vi "RT Data processing loop.vi"(9 "Data":T1={"Parameters"={"FPGA Ref"=refnum, "data stream"={"data writer name"="error writer", "NS write buffer size"=16, "NS Buffer length"=0}, "FIFO Depth"=0, "Channel controls"={"FIFO channel count"=0, "active indices"=[], "active channels"=0, "channelScaling"=[], "scanivalveCount"=0, "channels"=[]}, "safetyChannels"={"oilP"=0, "airP"=0, "water"=0, "channelLimits"=[]}, "speedChannel"=0, "maxSpeedLimit"=0.0, "Torque"={"fixedOffset"=0.0, "filter"=FALSE, "fallingEdge"=FALSE, "swapEncoders"=FALSE}}, "Variables"={"Intermediary buffer"=[], "buffer position"=0, "write loop counter"=0, "NS write trigger"=0, "NS Connection status"=FALSE, "waiting for NS"=FALSE, "labAmbient"={"pressure"=0.0, "temperature"=0.0}, "scanivalvePorts"=[], "scanivalvePressures"=[], "data stream"="", "activeChannelLimitIndex"=[], "runningSpeedLimit"=0.0, "speedChannelIndex"=0, "Interlocks"={"gearboxOil"=FALSE, "bearingOil"=FALSE, "gearboxAir"=FALSE}, "interlockChannels"={"gearboxOil"=0, "bearingOil"=0, "air"=0}, "limitStates"=[]}}, 11 "RT Queues":T8) -> ()   [LabVIEW 2018]
uses:
  Type Defs/Queues cluster.ctl
  ICL-LabVIEW_General/Message Scheduler/message scheduler.lvclass
  Type Defs/Data processing loop data.ctl
  Type Defs/FPGA reference.ctl
  PC/type defs/channelControl.ctl
  Type Defs/channelScalingTypes.ctl
  Type Defs/scalingMethods.ctl
  ICL-LabVIEW_General/data channels/parent class/Data Channel.lvclass
  PC/type defs/channelLimitControl.ctl
  PC/type defs/limitActions.ctl
  ICL-LabVIEW_General/data channels/parent class/Data Channel.lvclass/Data Channel.ctl
  <vilib>/dex/Flush And Wait Empty Condition.ctl
  Queue VIs/De-queue RT data element.vi
  Queue VIs/En-queue RT data element.vi
  Queue VIs/En-queue RT FIFO element.vi
  <vilib>/Utility/error.llb/Error Cluster From Error Code.vi
  <vilib>/rvi/errors/niLvFpgaAdjustHostInterfaceError.vi
  Queue VIs/Close RT data queue.vi
  <vilib>/rvi/interface/nirviReadWriteControl/nirviReadWriteControl.xnode
  FPGA Bitfiles/CompressorRigV2_CompressorFPGA_FPGAMainV3_7sPRekuravM.lvbitx
  NiFpgaLv.dll
panel:
  out "# elements in queue":i32
  out "Iteration Duration":i64[](array[numeric]) caption="Iteration Duration (max 10)"
  out "Processor resources low":bool
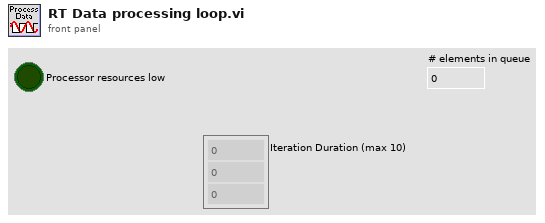
[diagram p1: front panel]
types:
  T1 = typedef "Data processing loop data.ctl" = cluster{"Parameters":cluster{"FPGA Ref":T2, "data stream":cluster{"data writer name":string, "NS write buffer size":i32, "NS Buffer length":u32}, "FIFO Depth":u32, "Channel controls":cluster{"FIFO channel count":i32, "active indices":i16[], "active channels":i32, "channelScaling":T3[], "scanivalveCount":i32, "channels":refnum<class "Data Channel.lvclass">[]}, "safetyChannels":cluster{"oilP":u16, "airP":u16, "water":u16, "channelLimits":T6[]}, "speedChannel":i32, "maxSpeedLimit":dbl, "Torque":cluster{"fixedOffset":dbl, "filter":bool, "fallingEdge":bool, "swapEncoders":bool}}, "Variables":cluster{"Intermediary buffer":dbl[][], "buffer position":u32, "write loop counter":u16, "NS write trigger":u32, "NS Connection status":bool, "waiting for NS":bool, "labAmbient":cluster{"pressure":dbl, "temperature":dbl}, "scanivalvePorts":u16[], "scanivalvePressures":dbl[], "data stream":refnum<k21>, "activeChannelLimitIndex":u16[], "runningSpeedLimit":dbl, "speedChannelIndex":i32, "Interlocks":cluster{"gearboxOil":bool, "bearingOil":bool, "gearboxAir":bool}, "interlockChannels":cluster{"gearboxOil":i32, "bearingOil":i32, "air":i32}, "limitStates":cluster{"warn":bool, "alarm":bool}[]}}
  T2 = typedef "FPGA reference.ctl" = refnum<k20>
  T3 = typedef "channelControl.ctl" = cluster{"index":u16, "active":bool, "channelType":T4, "module":u16, "terminal":u16, "channelName":string, "scalingMethod":T5, "scalingParameters":dbl[], "scaledUnits":string, "tempOffset":dbl}
  T4 = typedef "channelScalingTypes.ctl" = enum16{"calculation", "measurement", "scanivalve", "output", "digital"}
  T5 = typedef "scalingMethods.ctl" = enum16{"none", "linear", "thermocouple", "polynomial", "encoder", "RTD"}
  T6 = typedef "channelLimitControl.ctl" = cluster{"channelID":u16, "Enabled":bool, "warnValue":dbl, "limitValue":dbl, "Invert":bool, "limitAction":T7}
  T7 = typedef "limitActions.ctl" = enum16{"stop", "shutdown", "ignore"}
  T8 = typedef "Queues cluster.ctl" = cluster{"RT Message":refnum<queue>, "RT Comms":refnum<queue>, "RT Data":refnum<queue>, "RT FIFO":refnum<queue>, "message scheduler":refnum<class "message scheduler.lvclass">}
  T9 = typedef "Flush And Wait Empty Condition.ctl" = u8
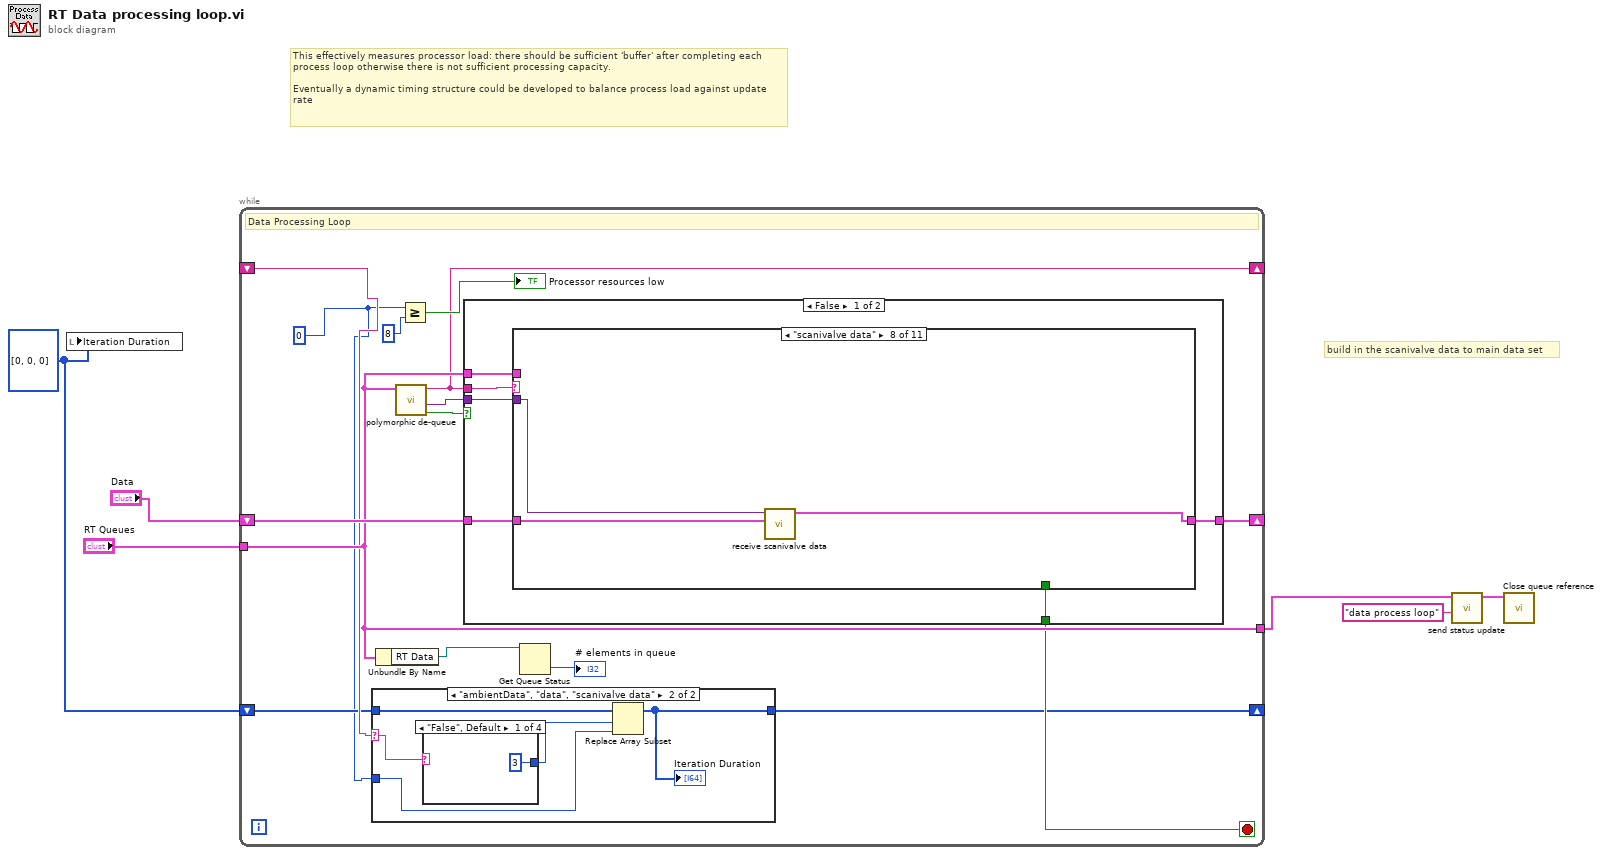
[diagram p0: block diagram]
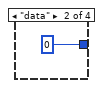
[diagram p3: hidden frame]
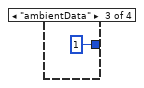
[diagram p4: hidden frame]
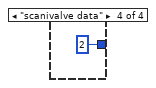
[diagram p5: hidden frame]
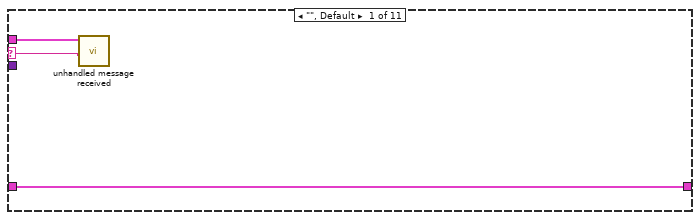
[diagram p6: hidden frame]
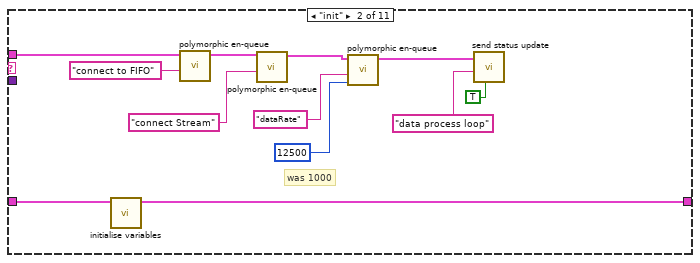
[diagram p7: hidden frame]
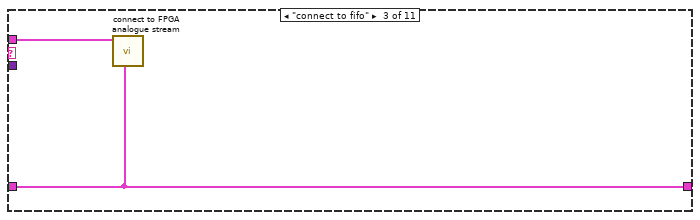
[diagram p8: hidden frame]
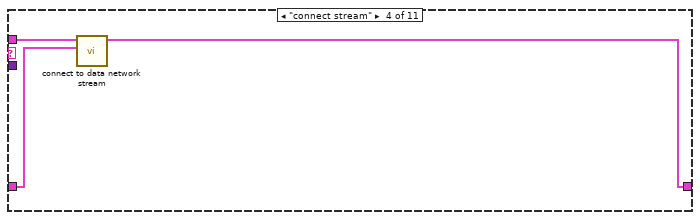
[diagram p9: hidden frame]
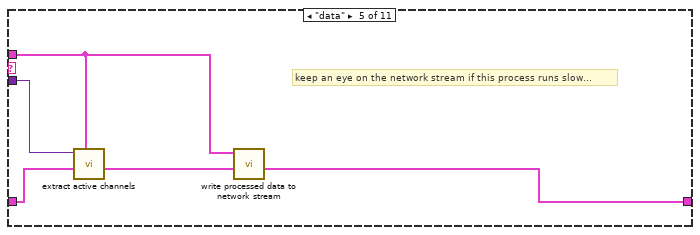
[diagram p10: hidden frame]
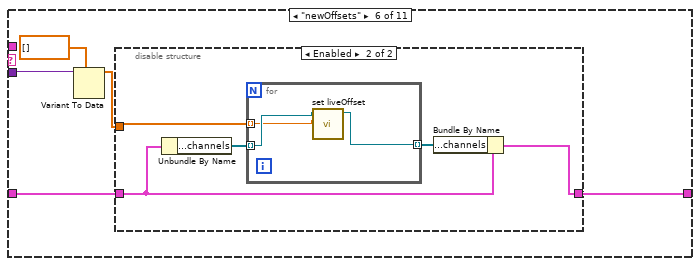
[diagram p11: hidden frame]
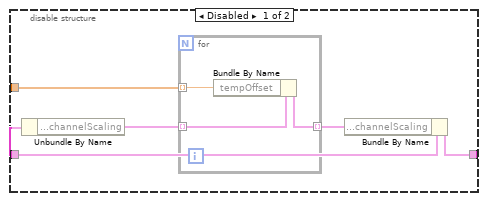
[diagram p12: hidden frame]
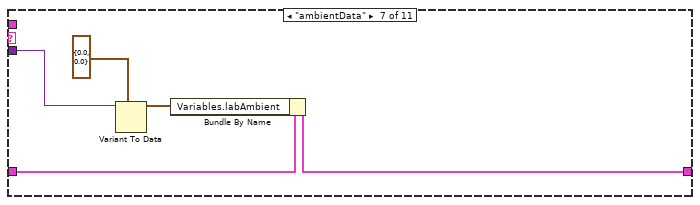
[diagram p13: hidden frame]
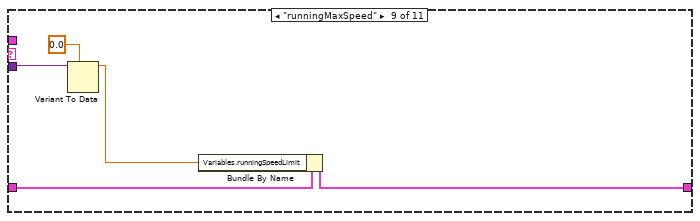
[diagram p14: hidden frame]
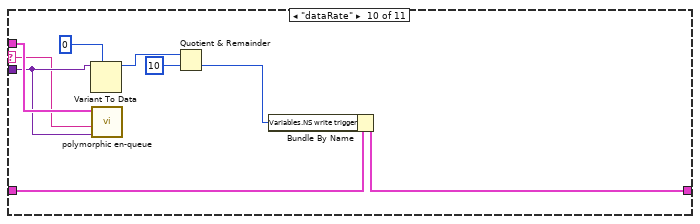
[diagram p15: hidden frame]
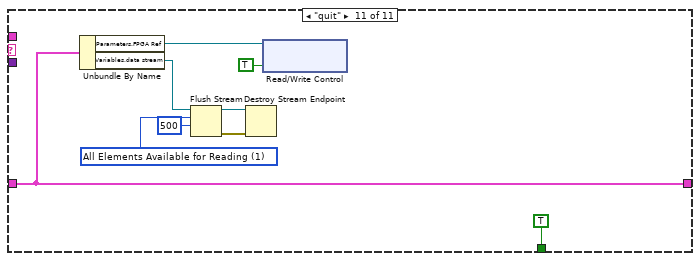
[diagram p16: hidden frame]
diagram:
  w1 = i64[] [0, 0, 0] ("Iteration Duration")
  # "build in the scanivalve data to main data set"
  # "This effectively measures processor load: there should be sufficient 'buffer' after completing each process loop otherwise there is not sufficient processing capacity.\n\nEventually a dynamic timing structure could be developed to balance process load against update rate"
  n1 = local write "Iteration Duration"(w1) -> ()
  n2 = while {
    tunnel: "RT Queues" -> [w15]
    tunnel: [w15] -> w4
    shift-right: [w20] -> _
    shift-left: "Data" -> [w19]
    shift-right: [w8] -> _
    shift-left: w1 -> [w9]
    shift-right: [w11] -> _
    shift-left: _ -> [w10]
    stop <- w12 stop-if-true
    w7 = i64 0 ("x")
    # "Data Processing Loop"
    n3 = case shown="\"ambientData\", \"data\", \"scanivalve data\"" w10 {
      selector: w10 -> [_ w26]
      tunnel: w9 -> [w22 w27]
      tunnel: [w22 w23] -> w8
      tunnel: w7 -> [_ w25]
      frame "", Default {
      }
      frame "ambientData", "data", "scanivalve data" {
        n4 = case shown="\"False\", Default" w26 {
          tunnel: [3 0 1 2] -> w24
          frame "False", Default {
          }
          frame "data" {
          }
          frame "ambientData" {
          }
          frame "scanivalve data" {
          }
        }
        n5 = Replace Array Subset(array=w27, new element=w25, index=w24) -> (w23:i64[])
        "Iteration Duration" <- w23
      }
    }
    n6 = Unbundle By Name(w15) -> ("RT Data"=w14:refnum<queue>)
    n7 = call-poly "polymorphic de-queue.vi"("RT Queues"=w15) -> ("timed out?"=w16:bool, "Data"=w21:variant, "Message"=w11:string)  [unwired: 8 in]
    n8 = Greater Or Equal?(x=w7, y=i64 8) -> (x >= y?=→"Processor resources low":bool)
    n9 = case shown="False" w16 {
      tunnel: w11 -> [w37 _]
      tunnel: w21 -> [w36 _]
      tunnel: w15 -> [w35 _]
      tunnel: [w34 w115] -> w20
      tunnel: w19 -> [w33 w115]
      tunnel: [w32 _] -> w12
      frame False {
        n10 = case shown="\"scanivalve data\"" w37 {
          selector: w37 -> [w38 _ _ _ _ _ _ _ _ w97 _]
          tunnel: w36 -> [_ _ _ _ w62 w65 w87 w91 w94 w98 _]
          tunnel: w35 -> [w39 w52 w54 w55 w58 _ _ _ _ w99 _]
          tunnel: [w40 w45 w53 w56 w59 w67 w85 w89 w95 w103 w114] -> w34
          tunnel: w33 -> [w40 w46 w53 w57 w61 w66 w88 w90 w96 w105 w114]
          tunnel: [_ _ _ _ _ _ _ _ _ _ TRUE] -> w32
          frame "", Default {
            n11 = call "unhandled message received.vi"("unhandled message"=w38, "RT Queues"=w39) -> ()  [unwired: 10 in]
          }
          frame "init" {
            # "was 1000"
            n12 = call "initialise variables.vi"("Data in"=w46) -> ("Data out"=w45:T1)  [unwired: 10 in]
            n13 = call-poly "polymorphic en-queue.vi"("Message"="connect to FIFO", "RT Queues"=w52) -> ("RT Queues out"=w50:T8)  [unwired: 7 in, 2 out]
            n14 = call-poly "polymorphic en-queue.vi"("Message"="connect Stream", "RT Queues"=w50) -> ("RT Queues out"=w44:T8)  [unwired: 7 in, 2 out]
            n15 = call-poly "polymorphic en-queue.vi"("Data"=u16 12500, "Message"="dataRate", "RT Queues"=w44) -> ("RT Queues out"=w43:T8)  [unwired: 6 in, 2 out]
            n16 = call "send status update.vi"("status (F)"=TRUE, "subject"="data process loop" ("Message"), "RT Queues"=w43) -> ()  [unwired: 8 in, 1 out]
          }
          frame "connect to fifo" {
            n17 = call "connect to FPGA analogue stream.vi"("Data"=w53, "RT Queues"=w54) -> ()  [unwired: 10 in]
          }
          frame "connect stream" {
            n18 = call "connect to data network stream.vi"("Data in"=w57, "RT Queues"=w55) -> ("Data out"=w56:T1)  [unwired: 9 in]
          }
          frame "data" {
            # "keep an eye on the network stream if this process runs slow..."
            n19 = call "extract active channels.vi"("RT Queues"=w58, "Data"=w61, "Data in"=w62) -> ("Data out"=w60:T1)  [unwired: 7 in, 1 out]
            n20 = call "write processed data to network stream.vi"("Data"=w60, "RT Queues"=w58) -> ("Data out"=w59:T1)  [unwired: 9 in]
          }
          frame "newOffsets" {
            n21 = Variant To Data(type=dbl[] [] ("tempOffset"), Variant=w65) -> (data=w63:dbl[])  [unwired: 1 in, 1 out]
            n22 = disable-structure shown="Enabled" {
              disable-tunnel: [w72 w80] -> w67
              disable-tunnel: w66 -> [w71 w79]
              disable-tunnel: w63 -> [w68 w77]
              frame Disabled {
                n23 = Unbundle By Name(w71) -> ("Parameters.Channel controls.channelScaling"=w69:T3[])
                n24 = for {
                  tunnel: [w74] -> w70 mode=indexing
                  tunnel: w69 -> [w75] mode=indexing
                  tunnel: w68 -> [w73] mode=indexing
                  n25 = Bundle By Name(cluster=w75, "tempOffset"=w73) -> (w74:T3)
                }
                n26 = Bundle By Name(cluster=w71, "Parameters.Channel controls.channelScaling"=w70) -> (w72:T1)
              }
              frame Enabled {
                n27 = Unbundle By Name(w79) -> ("Parameters.Channel controls.channels"=w78:refnum<class "Data Channel.lvclass">[])
                n28 = for {
                  tunnel: w78 -> [w83] mode=indexing
                  tunnel: w77 -> [w82] mode=indexing
                  tunnel: [w81] -> w76 mode=indexing
                  n29 = call "set liveOffset.vi"("liveOffset"=w82, "Data Channel in"=w83) -> ("Data Channel out"=w81:refnum<class "Data Channel.lvclass">)  [unwired: 9 in]
                }
                n30 = Bundle By Name(cluster=w79, "Parameters.Channel controls.channels"=w76) -> (w80:T1)
              }
            }
          }
          frame "ambientData" {
            n31 = Variant To Data(type=cluster{"pressure":dbl, "temperature":dbl} {"pressure"=0.0, "temperature"=0.0} ("labAmbient"), Variant=w87) -> (data=w84:cluster{"pressure":dbl, "temperature":dbl})  [unwired: 1 in, 1 out]
            n32 = Bundle By Name(cluster=w88, "Variables.labAmbient"=w84) -> (w85:T1)
          }
          frame "scanivalve data" {
            n33 = call "receive scanivalve data.vi"("Data in"=w90, "Data"=w91) -> ("Data out"=w89:T1)  [unwired: 9 in]
          }
          frame "runningMaxSpeed" {
            n34 = Variant To Data(type=0.0 ("Variables.runningSpeedLimit"), Variant=w94) -> (data=w93:dbl)  [unwired: 1 in, 1 out]
            n35 = Bundle By Name(cluster=w96, "Variables.runningSpeedLimit"=w93) -> (w95:T1)
          }
          frame "dataRate" {
            n36 = Variant To Data(type=u16 0, Variant=w98) -> (data=w101:u16)  [unwired: 1 in, 1 out]
            n37 = call-poly "polymorphic en-queue.vi"("Data"=w98, "Message"=w97, "RT Queues"=w99) -> ()  [unwired: 6 in, 3 out]
            n38 = Quotient & Remainder(x=w101, y=u16 10) -> (floor(x/y)=w102:u16)  [unwired: 1 out]
            n39 = Bundle By Name(cluster=w105, "Variables.NS write trigger"=w102) -> (w103:T1)
          }
          frame "quit" {
            w108 = T9 1 items=["All Elements Read From Stream", "All Elements Available for Reading"] ("wait condition")
            n40 = Unbundle By Name(w114) -> ("Parameters.FPGA Ref"=w113:T2, "Variables.data stream"=w112:refnum<k21>)
            n41 = Flush Stream(9:500 ("timeout in ms (-1)"), 10:w108, 11:w112) -> (0:w111:errorcluster, 3:w110:refnum<k21>)  [unwired: 1 in, 1 out]
            n42 = Destroy Stream Endpoint(8:w111, 11:w110) -> ()  [unwired: 1 out]
            n43 = xnode "Read/Write Control"("FPGA VI Reference In"=w113, "Stop acquire"=TRUE) -> ()  [unwired: 1 in, 2 out]
          }
        }
      }
      frame True {
      }
    }
    n44 = Get Queue Status(queue=w14) -> (# elements in queue=→"# elements in queue":i32)  [unwired: 2 in, 7 out]
  }
  n45 = call "send status update.vi"("subject"="data process loop" ("Message"), "RT Queues"=w4) -> ("RT Queues out"=w3:T8)  [unwired: 9 in]
  n46 = call-poly "Close queue reference.vi"("RT Queues"=w3) -> ()  [unwired: 11 in]
